vi "Configure Channel Characteristics Core.vi"(0 "IVI_Scope in":refnum<class "IVI_Scope.lvclass">, 5 "channel name (\"CHANNEL1\")":string="CHANNEL1", 7 "input impedance (1.0E+6 ohms)":dbl[unit]=1000000.0 format="%.2e", 9 "max input frequency (1.0E+6 Hz)":dbl[unit]=1000000.0 format="%.2e", 11 "error in (no error)":errorcluster) -> (4 "IVI_Scope out":refnum<class "IVI_Scope.lvclass">, 15 "error out":errorcluster)   [LabVIEW 2016, in "IVI_Scope.lvlib" / "IVI_Scope.lvclass"]
doc: "This VI configures the properties that control the electrical characteristics of the channel. These properties are the input impedance and the maximum frequency of the input signal."
uses:
  IVI_Scope.lvclass
  IVI_Scope.lvclass/IVI_Scope.ctl
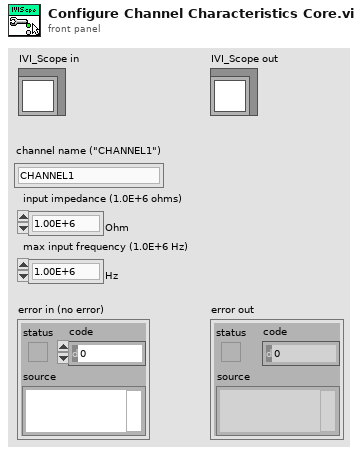
[diagram p1: front panel]
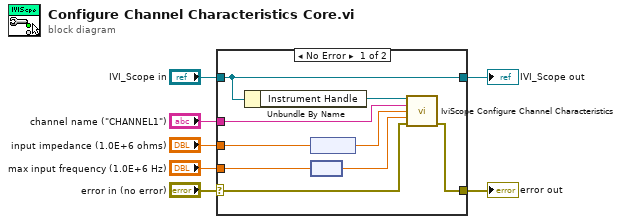
[diagram p0: block diagram]
diagram:
  n1 = case shown="No Error" "error in (no error)" {
    selector: "error in (no error)" -> [w14 w18]
    tunnel: [w13 w18] -> w6
    tunnel: [w16 w17] -> w4
    tunnel: "IVI_Scope in" -> [w16 w17]
    tunnel: "channel name (\"CHANNEL1\")" -> [w12 _]
    tunnel: "input impedance (1.0E+6 ohms)" -> [w11 _]
    tunnel: "max input frequency (1.0E+6 Hz)" -> [w10 _]
    frame No Error {
      n2 = Unbundle By Name(w16) -> ("Instrument Handle"=w15:refnum<k15>)
      n3 = node(w11) -> (w8:dbl)
      n4 = node(w10) -> (w9:dbl)
      n5 = call <vilib>:"IviScope Configure Channel Characteristics.vi"("instrument handle"=w15, "channel name (\"CHANNEL1\")"=w12, "input impedance (1.0E+6 ohms)"=w8, "max input frequency (1.0E+6 Hz)"=w9, "error in (no error)"=w14) -> ("error out"=w13:errorcluster)  [unwired: 9 in, 1 out]
    }
    frame Error {
    }
  }
  "error out" <- w6
  "IVI_Scope out" <- w4
